vi "更新主程序.vi"() -> ()   [LabVIEW 2016]
uses:
  <vilib>/FTP/NI_FTP.lvlib
  update.lvlib
panel:
  in  "取消按钮":bool
  out "command":string caption="命令"
  out "last status string":string caption="最近状态字符串"
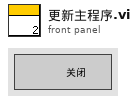
[diagram p1: front panel]
types:
  T1 = cluster{"remote path":string, "local path":path, "binary":bool}
  T2 = cluster{"remote path":string, "local path":path, "binary":bool}[]
  T3 = enum32{"invalid app kind", "Development System", "Run Time System", "Student Edition", "Embedded LabVIEW", "Evaluation", "Custom"}
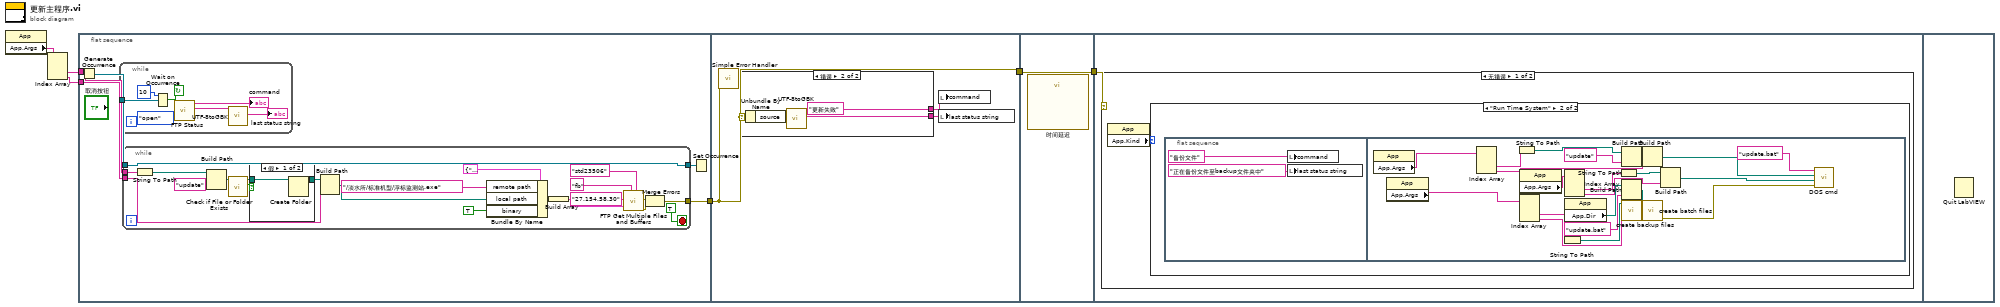
[diagram p0: block diagram]
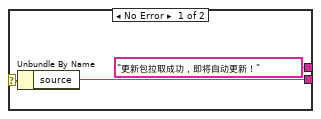
[diagram p3: hidden frame]
diagram:
  n1 = property class="App"() -> ("App.Args"=w3:string[])  [unwired: 2 in, 2 out]
  n2 = Index Array(array=w3) -> (element #2=w1:string, element #3=w2:string)  [unwired: 3 in, 1 out]
  n3 = flat-sequence {
    tunnel: [w9] -> w6
    tunnel: w2 -> [w8]
    tunnel: w1 -> [w7]
    tunnel: w6 -> [w44]
    tunnel: [w44] -> w5
    tunnel: w5 -> [w54]
    tunnel: [w54] -> w4
    tunnel: w4 -> [w55]
    frame #0 {
      n4 = Generate Occurrence() -> (w10:refnum<k4>)
      n5 = while {
        tunnel: w10 -> [w42]
        stop <- w40 continue-if-true
        n6 = Wait on Occurrence(2:w42, 3:10 ("毫秒超时(-1)")) -> (0:w40:bool)  [unwired: 1 in]
        n7 = call "FTP Status"("window"=enum16{"nothing", "open", "close"}."open") -> ("last status string"=w39:string, "command"=→"command":string)  [unwired: 9 in]
        n8 = call "UTF-8toGBK.vi"("UTF-8"=w39) -> ("GBK"=→"last status string":string)  [unwired: 9 in, 1 out]
      }
      n9 = while {
        tunnel: [w32] -> w11
        tunnel: w10 -> [w32]
        tunnel: [w31] -> w9
        tunnel: w8 -> [w14]
        tunnel: w7 -> [w13]
        stop <- TRUE stop-if-true
        n10 = String To Path(string=w13) -> (path=w12:path)
        n11 = Build Path(base path=w12, name or relative path="update" ("名称或相对路径")) -> (appended path=w22:path)
        n12 = call <vilib>:"Check if File or Folder Exists.vi"("path"=w22) -> ("file or folder exists?"=w21:bool, "dup path"=w20:path)  [unwired: 8 in, 1 out]
        n13 = case shown="假" w21 {
          tunnel: w20 -> [w35 w36]
          tunnel: [w34 w36] -> w19
          frame False {
            n14 = Create Folder(path (use dialog)=w35) -> (created path=w34:path)  [unwired: 2 in, 2 out]
          }
          frame True {
          }
        }
        n15 = Build Path(base path=w19, name or relative path=w14) -> (appended path=w24:path)
        n16 = Bundle By Name(cluster=T1 {"remote path"="", "local path"=path "", "binary"=FALSE} ("transfer spec"), "remote path"="/淡水所/标准机型/浮标监测站.exe", "local path"=w24, "binary"=TRUE) -> (w25:T1)
        n17 = Build Array(w25) -> (w26:T2)
        n18 = call <vilib>:"FTP Get Multiple Files and Buffers.vi"("password"="std23506", "user"="fb", "file specifications"=w26, "host"="27.154.58.30") -> ("error out"=w15:errorcluster, "file errors"=w16:errorcluster[])  [unwired: 5 in, 1 out]
        n19 = Merge Errors(w16, w15) -> (w31:errorcluster)
      }
      n20 = Set Occurrence(w11) -> ()
    }
    frame #1 {
      n21 = call <vilib>:"Simple Error Handler.vi"("error in (no error)"=w44) -> ()  [unwired: 4 in, 5 out]
      n22 = case shown="错误" w44 {
        selector: w44 -> [w48 w53]
        tunnel: ["更新包拉取成功，即将自动更新！" ("command") "更新失败" ("command")] -> w46
        tunnel: [w47 w50] -> w45
        frame No Error {
          n23 = Unbundle By Name(w48) -> ("source"=w47:string)
        }
        frame Error {
          n24 = Unbundle By Name(w53) -> ("source"=w51:string)
          n25 = call "UTF-8toGBK.vi"("UTF-8"=w51) -> ("GBK"=w50:string)  [unwired: 9 in, 1 out]
        }
      }
      n26 = local write "command"(w46) -> ()
      n27 = local write "last status string"(w45) -> ()
    }
    frame #2 {
      n28 = call "时间延迟"() -> ()  [unwired: 11 in, 1 out]
    }
    frame #3 {
      n29 = case shown="无错误" w55 {
        frame No Error {
          n30 = property class="App"() -> ("App.Kind"=w56:T3)  [unwired: 2 in, 2 out]
          n31 = case shown="\"Run Time System\"" w56 {
            frame "invalid app kind", Default {
            }
            frame "Run Time System" {
              n32 = flat-sequence {
                frame #0 {
                  n33 = local write "command"("备份文件" ("command")) -> ()
                  n34 = local write "last status string"("正在备份文件至backup文件夹中" ("last status string")) -> ()
                }
                frame #1 {
                  n35 = property class="App"() -> ("App.Args"=w68:string[])  [unwired: 2 in, 2 out]
                  n36 = property class="App"() -> ("App.Args"=w75:string[])  [unwired: 2 in, 2 out]
                  n37 = Index Array(array=w68) -> (element #2=w69:string, element #3=w64:string)  [unwired: 3 in, 1 out]
                  n38 = String To Path(string=w69) -> (path=w67:path)
                  n39 = property class="App"() -> ("App.Args"=w71:string[])  [unwired: 2 in, 2 out]
                  n40 = Index Array(array=w75) -> (element #2=w78:string, element #3=w76:string)  [unwired: 3 in, 1 out]
                  n41 = String To Path(string=w78) -> (path=w79:path)
                  n42 = Index Array(array=w71) -> (element #2=w62:string, element #3=w63:string)  [unwired: 3 in, 1 out]
                  n43 = property class="App"() -> ("App.Dir"=w74:path)  [unwired: 2 in, 2 out]
                  n44 = String To Path(string=w62) -> (path=w70:path)
                  n45 = Build Path(base path=w67, name or relative path="update" ("名称或相对路径")) -> (appended path=w65:path)
                  n46 = Build Path(base path=w74, name or relative path="update.bat" ("batch file name")) -> (appended path=w73:path)
                  n47 = call "create backup files.vi"("execute file name"=w76, "路径"=w79) -> ("error out"=w77:errorcluster)  [unwired: 9 in]
                  n48 = Build Path(base path=w65, name or relative path=w64) -> (appended path=w60:path)
                  n49 = call "create batch files.vi"("错误输入（无错误）"=w77, "Batch file"=w73) -> ("错误输出"=w80:errorcluster)  [unwired: 9 in]
                  n50 = Build Path(base path=w70, name or relative path=w63) -> (appended path=w59:path)
                  n51 = call "DOS cmd.vi"("错误输入（无错误）"=w80, 9:w59, 10:w60, "batch file"="update.bat" ("batch file name")) -> ()  [unwired: 7 in, 1 out]
                }
              }
            }
          }
        }
        frame Error {
        }
      }
    }
    frame #4 {
      n52 = Quit LabVIEW() -> ()  [unwired: 1 in]
    }
  }
